vi "set_params.vi"(8 "error in (no error)":errorcluster caption="entrée d'erreur (pas d'erreur)", 11 "NMF.lvclass 2":refnum<class "NMF.lvclass">) -> (0 "error out":errorcluster caption="sortie d'erreur", 3 "NMF.lvclass":refnum<class "NMF.lvclass">)   [LabVIEW 2020, in "NMF.lvclass"]
uses:
  NMF.lvclass
  NMF.lvclass/NMF.ctl
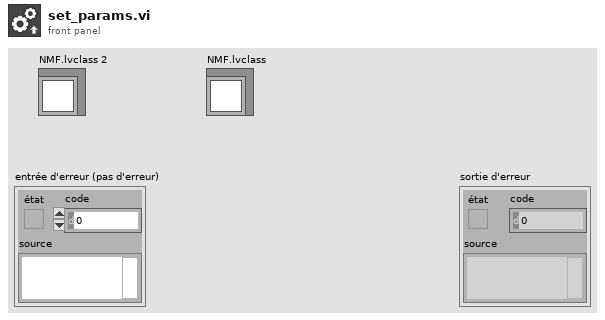
[diagram p1: front panel]
types:
  T1 = typedef "non_negative_matrix_factorization_params.ctl" = cluster{"n_components":cluster{"n_components_type":string, "n_components_int":dbl}, "init":string, "solver":string, "beta_loss":cluster{"beta_loss_type":string, "beta_loss_float":dbl}, "tol":dbl, "max_iter":dbl, "random_state":dbl, "alpha":dbl, "l1_ratio":dbl, "verbose":dbl, "shuffle":bool, "regularization":string}
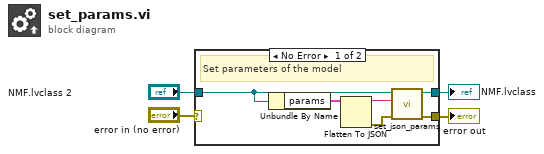
[diagram p0: block diagram]
diagram:
  n1 = case shown="No Error" "error in (no error)" {
    selector: "error in (no error)" -> [_ w12]
    tunnel: [w7 w12] -> w3
    tunnel: [w8 w11] -> w1
    tunnel: "NMF.lvclass 2" -> [w5 w11]
    frame No Error {
      # "Set parameters of the model"
      n2 = Unbundle By Name(w5) -> ("params"=w10:T1)
      n3 = Flatten To JSON(anything=w10) -> (JSON string=w9:string, 11:w6:errorcluster)  [unwired: 2 in]
      n4 = call-dynamic "set_json_params.vi"("error in (no error)"=w6, "params"=w9, "Model en entrée"=w5) -> ("error out"=w7:errorcluster, "Model en sortie"=w8:refnum<class "NMF.lvclass">)  [unwired: 7 in]
    }
    frame Error {
    }
  }
  "error out" <- w3
  "NMF.lvclass" <- w1
